vi "Place_Boxes.vi"(1 "Boxes Properties":T1[](array[typedef])) -> ()   [LabVIEW 2015]
uses:
  Controls/Box_Properties.ctl
  Controls/Box_Location.ctl
  Controls/Container_Properties.ctl
panel:
  out "Array":bool[][](array[boolean])
  out "Boxes Properties 2":T1[](array[typedef])
  out "Initialized Container":T3[](array[typedef])
  in  "Container Properties":T3[](array[typedef])
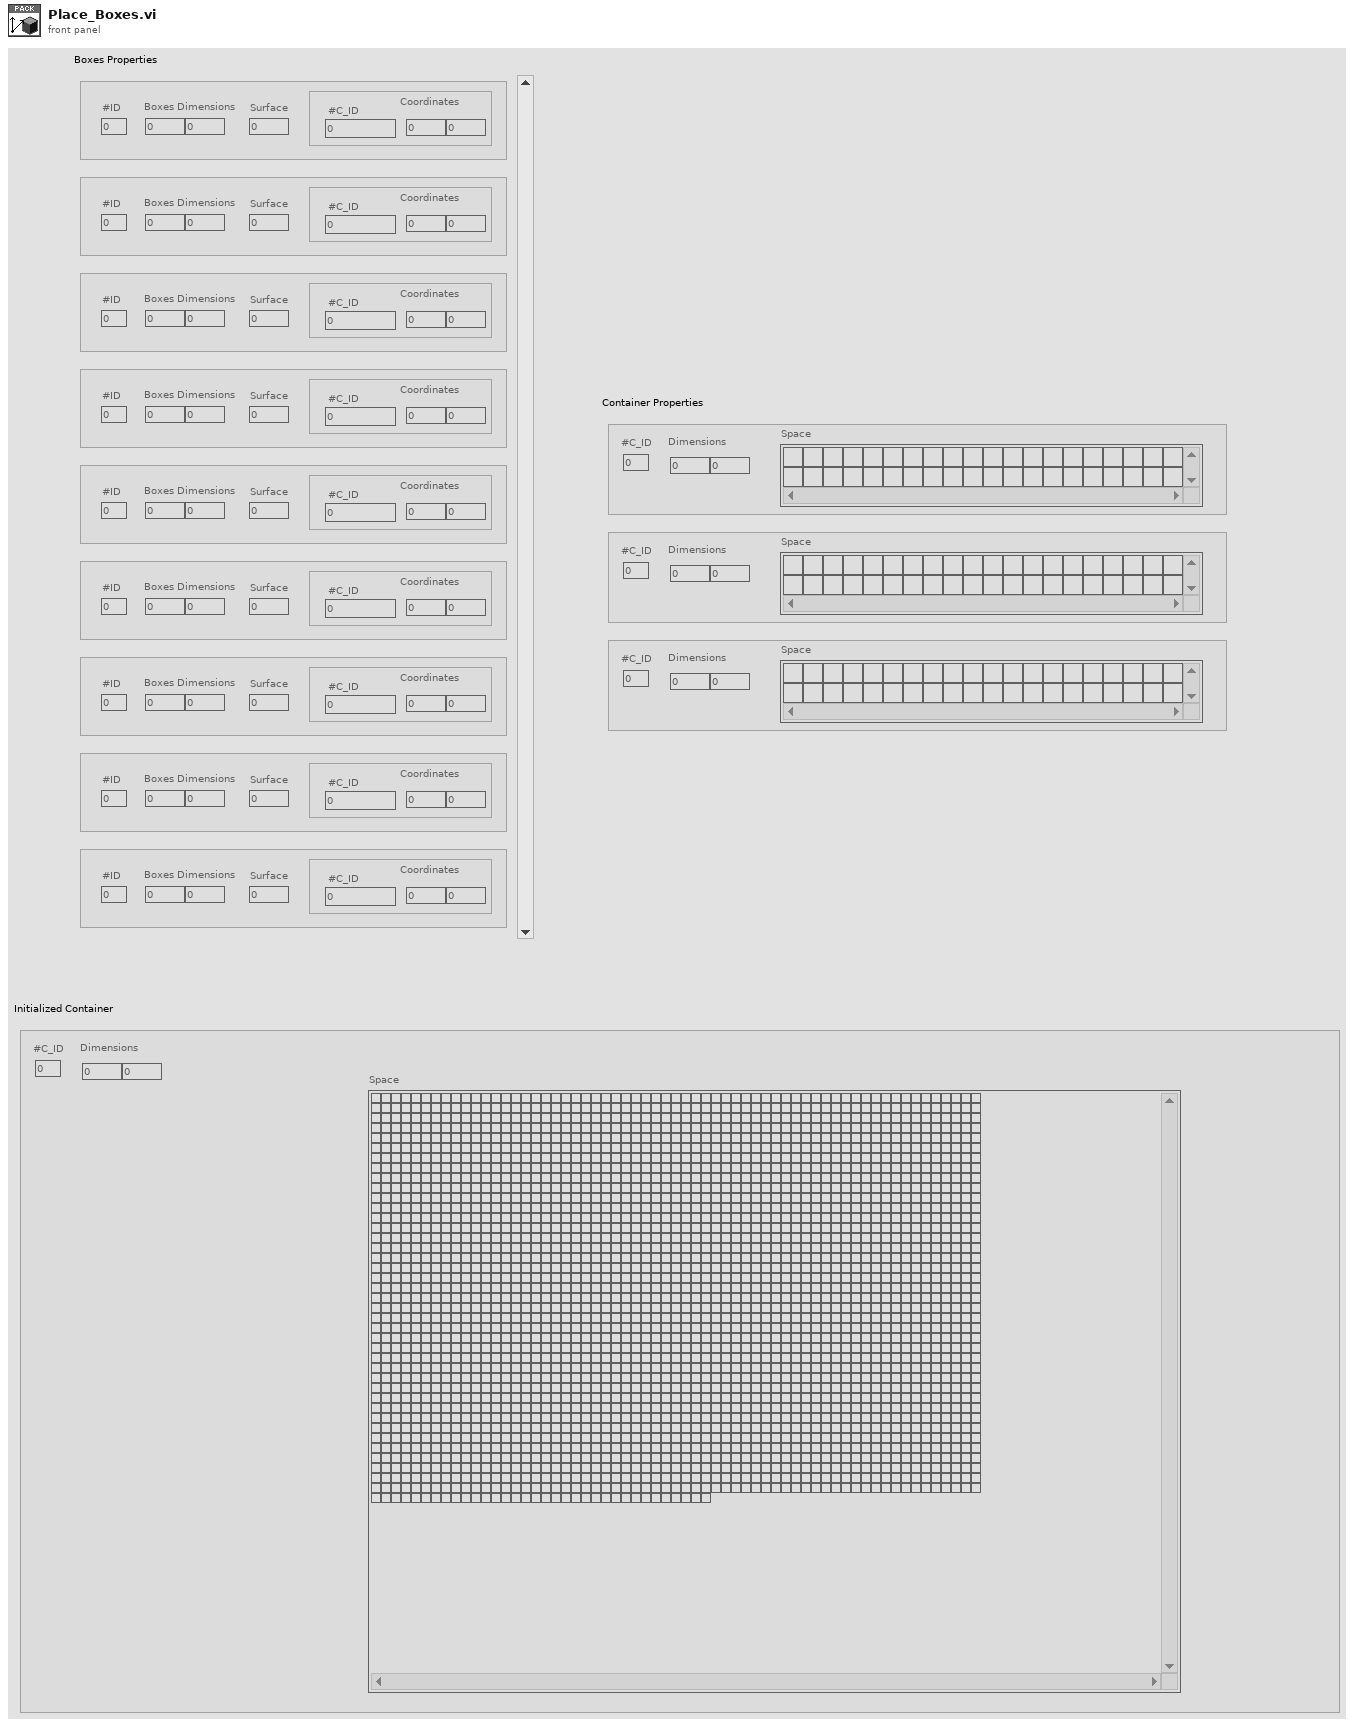
[diagram p1: front panel]
types:
  T1 = typedef "Box_Properties.ctl" = cluster{"Boxes Dimensions":dbl[], "Surface":dbl, "#ID":dbl, "Location":T2}
  T2 = typedef "Box_Location.ctl" = cluster{"#C_ID":dbl, "Coordinates":dbl[]}
  T3 = typedef "Container_Properties.ctl" = cluster{"#C_ID":dbl, "Dimensions":dbl[], "Space":bool[][]}
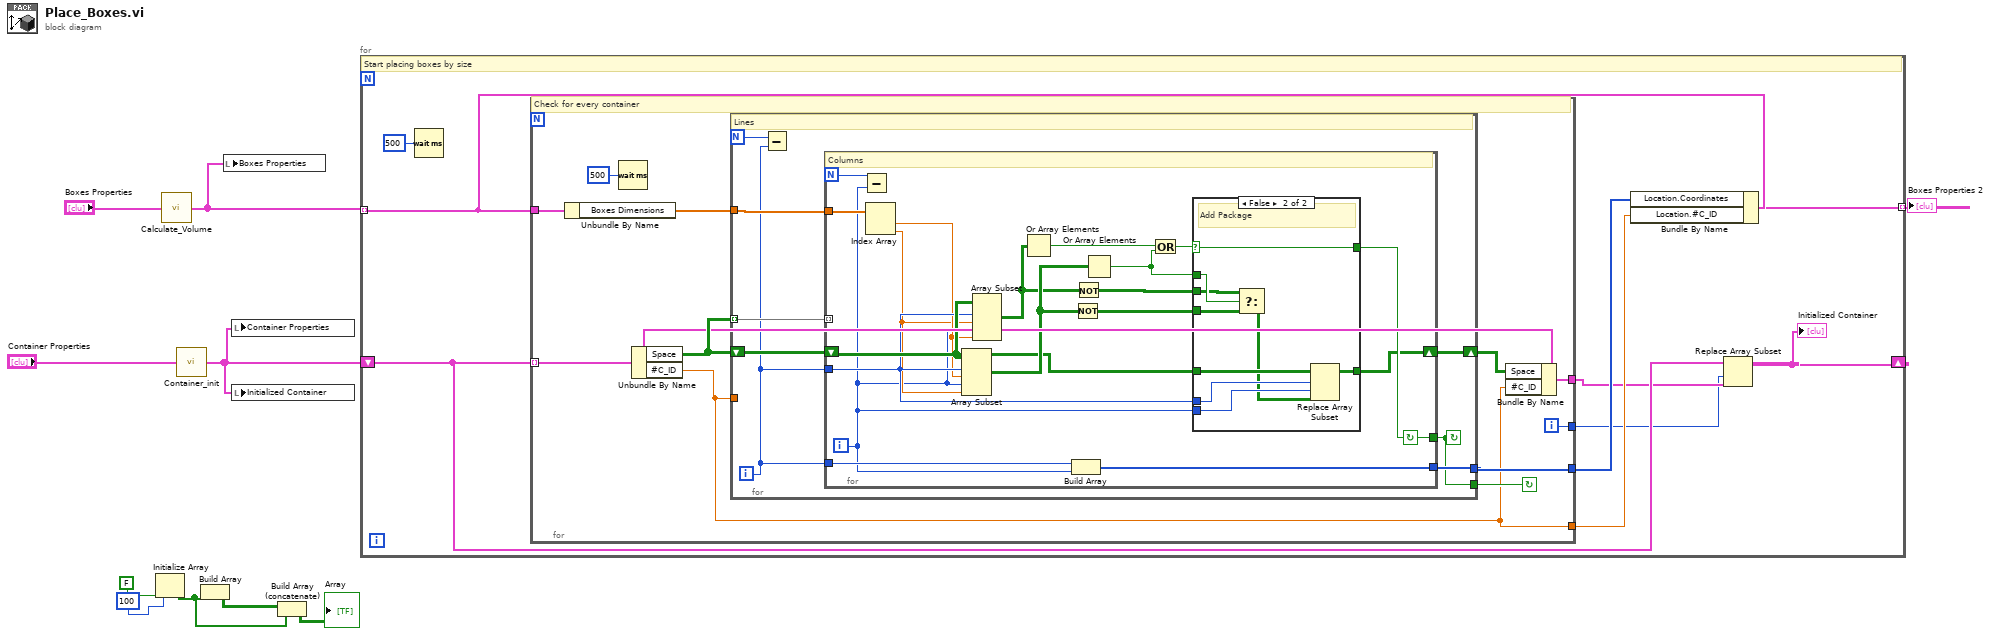
[diagram p0: block diagram]
diagram:
  n1 = Initialize Array(FALSE, 100 ("dimension size")) -> (w5:bool[])
  n2 = call "Calculate_Volume.vi"("Boxes Dimensions"="Boxes Properties") -> ("Sorted Boxes"=w1:T1[])
  n3 = call "Container_init.vi"("Container Properties"="Container Properties") -> ("Array"=w3:T3[])
  n4 = Build Array(w5, w5) -> (w6:bool[][])
  n5 = local write "Boxes Properties"(w1) -> ()
  n6 = local write "Container Properties"(w3) -> ()
  n7 = local write "Initialized Container"(w3) -> ()
  n8 = Build Array (concatenate)(w6, w5) -> (→"Array":bool[][])
  n9 = for {
    tunnel: w1 -> [w19] mode=indexing
    tunnel: [w18] -> w9 mode=indexing
    shift-right: [w11] -> _
    shift-left: w3 -> [w15]
    # "Start placing boxes by size"
    n10 = Wait (ms)(milliseconds to wait=u32 500) -> ()  [unwired: 1 out]
    n11 = for {
      tunnel: w15 -> [w21] mode=indexing
      tunnel: w19 -> [w30]
      tunnel: [w29] -> w17
      tunnel: [w25] -> w14
      tunnel: [w24] -> w16
      tunnel: [w23] -> w13
      i -> [w23]
      stop <- w28 continue-if-true
      # "Check for every container"
      n12 = Unbundle By Name(w30) -> ("Boxes Dimensions"=w20:dbl[])
      n13 = Wait (ms)(milliseconds to wait=u32 500) -> ()  [unwired: 1 out]
      n14 = Unbundle By Name(w21) -> ("Space"=w27:bool[][], "#C_ID"=w24:dbl)
      n15 = for {
        N -> [w32]
        tunnel: w24 -> [_]
        shift-right: [w37] -> w26
        shift-left: w27 -> [w38]
        tunnel: [w36] -> w29
        tunnel: [w35] -> w28
        tunnel: w27 -> [w34] mode=indexing
        tunnel: w20 -> [w33]
        i -> [w31]
        stop <- w35 continue-if-true
        # "Lines"
        n16 = Subtract(x=w32, y=w31) -> ()  [unwired: 1 out]
        n17 = for {
          N -> [w40]
          tunnel: w31 -> [w49]
          tunnel: [w56] -> w35
          shift-right: [w54] -> w37
          shift-left: w38 -> [w50]
          tunnel: w31 -> [w53]
          tunnel: [w52] -> w36
          tunnel: w34 -> [_] mode=indexing
          tunnel: w33 -> [w51]
          i -> [w39]
          stop <- w56 continue-if-true
          # "Columns"
          n18 = Subtract(x=w40, y=w39) -> ()  [unwired: 1 out]
          n19 = Index Array(array=w51) -> (element #1=w48:dbl, element #2=w47:dbl)  [unwired: 2 in]
          n20 = Array Subset(array=w50, index (row)=w49, length (row)=w48, index (col)=w39, length (col)=w47) -> (w55:bool[][])
          n21 = Array Subset(array=w50, index (row)=w49, length (row)=w47, index (col)=w39, length (col)=w48) -> (w42:bool[][])
          n22 = Or Array Elements(Boolean array=w42) -> (logical OR=w46:bool)
          n23 = Build Array(w53, w39) -> (w52:i32[])
          n24 = Not(x=w55) -> (.not. x?=w43:bool[][])
          n25 = Not(x=w42) -> (.not. x?=w41:bool[][])
          n26 = Or Array Elements(Boolean array=w55) -> (logical OR=w44:bool)
          n27 = Or(x=w46, y=w44) -> (x .or. y?=w45:bool)
          n28 = case shown="False" w45 {
            selector: w45 -> [w58 w66]
            tunnel: w50 -> [w57 w67]
            tunnel: [w58 w66] -> w56
            tunnel: w49 -> [_ w65]
            tunnel: w39 -> [_ w64]
            tunnel: w43 -> [_ w61]
            tunnel: [w57 w63] -> w54
            tunnel: w44 -> [_ w62]
            tunnel: w41 -> [_ w60]
            frame True {
            }
            frame False {
              # "Add Package"
              n29 = Select(t=w60, s=w62, f=w61) -> (s? t:f=w59:bool[][])
              n30 = Replace Array Subset(array=w67, new element=w59, index (row)=w65, index (col)=w64) -> (w63:bool[][])
            }
          }
        }
      }
      n31 = Bundle By Name(cluster=w21, "Space"=w26, "#C_ID"=w24) -> (w25:T3)
    }
    n32 = Bundle By Name(cluster=w19, "Location.Coordinates"=w17, "Location.#C_ID"=w16) -> (w18:T1)
    n33 = Replace Array Subset(array=w15, new element=w14, index=w13) -> (w11:T3[])
    "Initialized Container" <- w11
  }
  "Boxes Properties 2" <- w9
